vi "sub_main_state.vi"(8 "error in":errorcluster) -> (0 "error out":errorcluster)   [LabVIEW 2019]
uses:
  Ctrl/waypoint_buf.ctl
  Ctrl/state.ctl
  Ctrl/pid-in-params.ctl
  Ctrl/gps-databuf.ctl
panel:
  out "angle check":T1(graph)
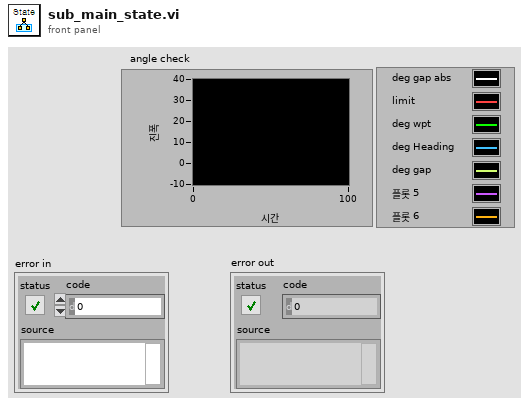
[diagram p1: front panel]
types:
  T1 = cluster{dbl, "adjust angle margin":dbl, "deg_waypoint":dbl, "Heading":dbl, dbl}
  T2 = typedef "waypoint_buf.ctl" = enum16{"clear", "write", "read"}
  T3 = typedef "state.ctl" = enum16{"init", "Test circular track", "start point", "start heading adjust", "wait before start", "stop point check", "stop point start", "end point", "entering ending point", "move", "move heading adjust"}
  T4 = typedef "pid-in-params.ctl" = enum16{"read", "write"}
  T5 = typedef "gps-databuf.ctl" = enum16{"read", "write"}
  T6 = cluster{"wpt group i":i32, "state total i":i32, "state main i":i32}
  T7 = cluster{"start point":cluster{"x":dbl, "y":dbl}, "stop point":cluster{"x":dbl, "y":dbl}}
  T8 = cluster{"lookahead pt n":dbl, "lookahead distance":dbl}
  T9 = cluster{"deg_agv-lookahead":dbl, "deg_waypoint":dbl, "deg_gap":dbl, "deg_target":dbl, "pid output":dbl, "dis-gap":dbl, "deg_agv-center":dbl}
  T10 = cluster{" turn angular speed":dbl, "move linear speed":dbl, "decrease factor linear speed":dbl, "adjust angle margin":dbl}
  T11 = cluster{"rawdata":string, "GPS Data":cluster{"Latitude":cluster{"Valid?":bool, "Latitude (Deg)":dbl}, "Longitude":cluster{"Valid?":bool, "Longitude (Deg)":dbl}, "Height":cluster{"Valid?":bool, "Height (m)":dbl}, "Undulation":cluster{"Valid?":bool, "Undulation(m)":dbl}, "North Vel":cluster{"Valid?":bool, "North Vel (m/s)":dbl}, "East Vel":cluster{"Valid?":bool, "East Vel (m/s)":dbl}, "Up Vel":cluster{"Valid?":bool, "Up Vel (m/s)":dbl}, "Roll":cluster{"Valid?":bool, "Roll (degrees)":dbl}, "Pitch":cluster{"Valid?":bool, "Pitch (degrees)":dbl}, "Azimuth":cluster{"Valid?":bool, "Azimuth (degrees)":dbl}, "Lat deviation":cluster{"Valid?":bool, "Lat deviation (m)":dbl}, "Long deviation":cluster{"Valid?":bool, "Long deviation (m)":dbl}, "Height deviation":cluster{"Valid?":bool, "Height deviation (m)":dbl}, "North vel deviation":cluster{"Valid?":bool, "North vel deviation (m/s)":dbl}, "East vel deviation":cluster{"Valid?":bool, "East vel deviation (m/s)":dbl}, "Up vel deviation":cluster{"Valid?":bool, "Up vel deviation (m/s)":dbl}, "Roll deviation":cluster{"Valid?":bool, "Roll deviation (degrees)":dbl}, "Pitch deviation":cluster{"Valid?":bool, "Pitch deviation (degrees)":dbl}, "Azimuth deviation":cluster{"Valid?":bool, "Azimuth deviation (degrees)":dbl}, "Ext sol status":cluster{"Valid?":bool, "Ext sol status":dbl}}, "Heading":dbl, "utm-1":cluster{"XN":dbl, "YE":dbl}}
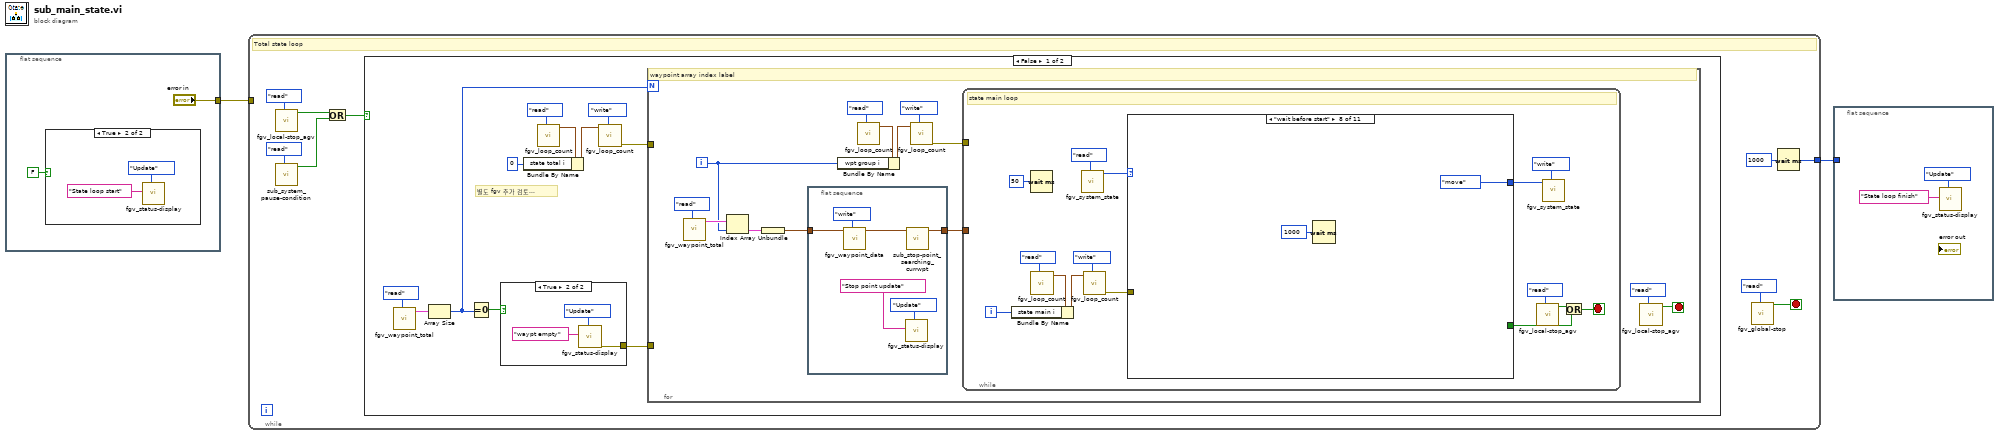
[diagram p0: block diagram]
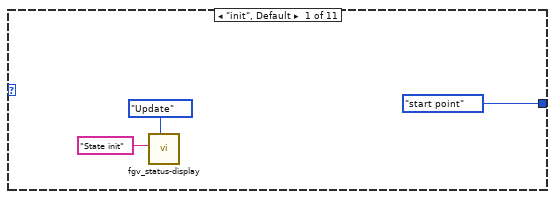
[diagram p4: hidden frame]
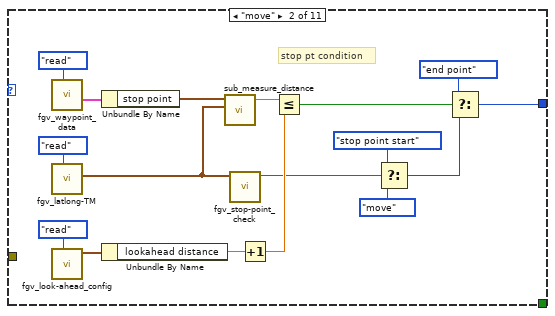
[diagram p5: hidden frame]
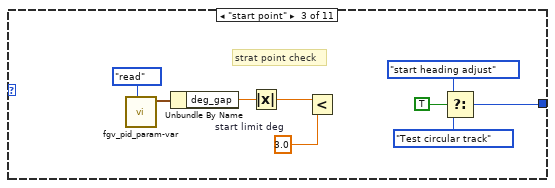
[diagram p6: hidden frame]
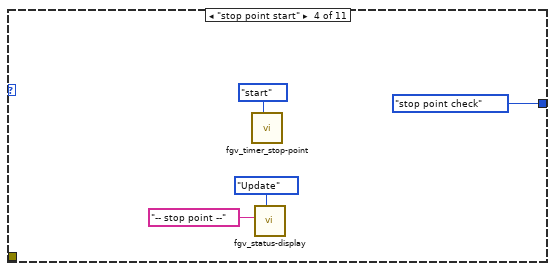
[diagram p7: hidden frame]
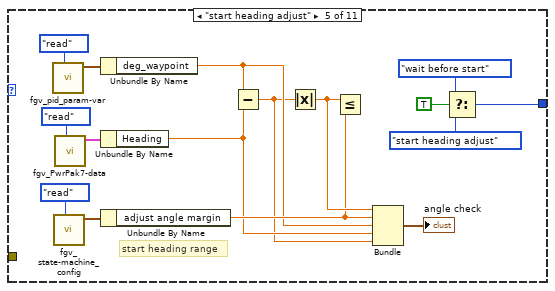
[diagram p8: hidden frame]
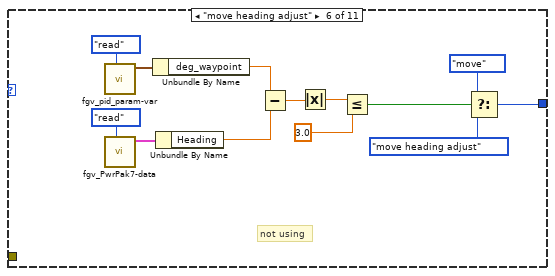
[diagram p9: hidden frame]
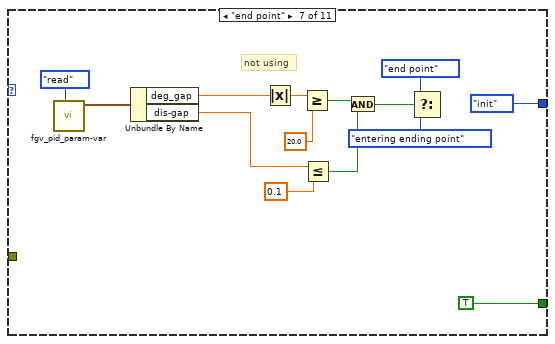
[diagram p10: hidden frame]
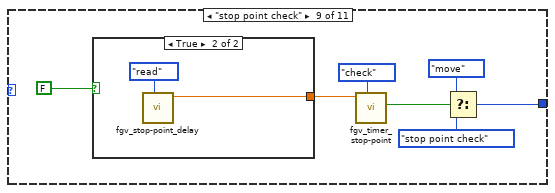
[diagram p11: hidden frame]
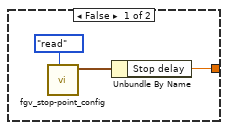
[diagram p12: hidden frame]
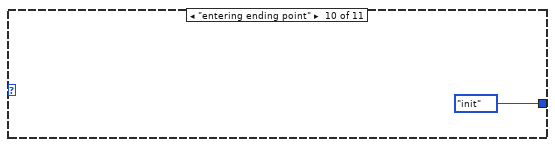
[diagram p13: hidden frame]
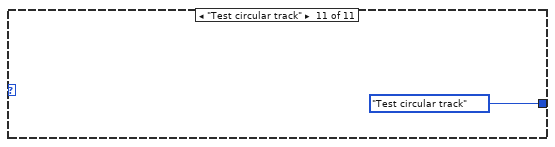
[diagram p14: hidden frame]
diagram:
  n1 = flat-sequence {
    tunnel: ["error in"] -> w2
    frame #0 {
      n2 = case shown="True" FALSE {
        frame False {
        }
        frame True {
          n3 = call "fgv_status-display.vi"("Mode"=enum16{"Initial", "Update", "Clear"}."Update", "title"="State loop start" ("String in 1")) -> ()  [unwired: 9 in, 1 out]
        }
      }
    }
  }
  n4 = while {
    tunnel: w2 -> [_]
    tunnel: [w14] -> w1
    stop <- w12 stop-if-true
    # "Total state loop"
    n5 = call "fgv_local-stop_agv.vi"("cmd"=enum16{"ini", "read", "stop"}."read") -> ("stop status"=w9:bool)  [unwired: 10 in]
    n6 = call "sub_system_pause-condition.vi"("cmd"=enum16{"pause", "go", "read"}."read") -> ("pause"=w7:bool)  [unwired: 10 in]
    n7 = Or(x=w9, y=w7) -> (x .or. y?=w8:bool)
    n8 = case shown="False" w8 {
      frame False {
        # "별도 fgv 추가 검토..."
        n9 = call "fgv_waypoint_total.vi"("cmd"=enum16{"write", "read"}."read") -> ("waypoint total out"=w24:cluster{"waypt":cluster{"X":dbl, "Y":dbl}[]}[])  [unwired: 10 in]
        n10 = Array Size(array=w24) -> (size(s)=w17:i32)
        n11 = Equal To 0?(x=w17) -> (x = 0?=w19:bool)
        n12 = case shown="True" w19 {
          tunnel: [_ w27] -> w26
          frame False {
          }
          frame True {
            n13 = call "fgv_status-display.vi"("Mode"=enum16{"Initial", "Update", "Clear"}."Update", "title"="waypt empty" ("String in 1")) -> ("error out"=w27:errorcluster)  [unwired: 9 in]
          }
        }
        n14 = call "fgv_loop_count.vi"("cmd"=enum16{"init", "read", "write"}."read") -> ("loop count out"=w21:T6)  [unwired: 9 in, 1 out]
        n15 = Bundle By Name(cluster=w21, "state total i"=0) -> (w20:T6)
        n16 = call "fgv_loop_count.vi"("cmd"=enum16{"init", "read", "write"}."write", "loop count in"=w20) -> ("error out"=w18:errorcluster)  [unwired: 8 in, 1 out]
        n17 = for {
          N: w17 -> [_]
          tunnel: w26 -> [_]
          tunnel: w18 -> [_]
          i -> [w32]
          stop <- w41 stop-if-true
          # "waypoint array index label"
          n18 = call "fgv_waypoint_total.vi"("cmd"=enum16{"write", "read"}."read") -> ("waypoint total out"=w33:cluster{"waypt":cluster{"X":dbl, "Y":dbl}[]}[])  [unwired: 10 in]
          n19 = Index Array(array=w33, index=w32) -> (element=w31:cluster{"waypt":cluster{"X":dbl, "Y":dbl}[]})
          n20 = Unbundle(w31) -> ("waypt"=w36:cluster{"X":dbl, "Y":dbl}[])
          n21 = flat-sequence {
            tunnel: w36 -> [w47]
            tunnel: [w43] -> w30
            frame #0 {
              n22 = call "fgv_waypoint_data.vi"("cmd"=waypoint_buf."write", "waypoint in"=w47) -> ("waypoint out"=w44:cluster{"x":dbl, "y":dbl}[])  [unwired: 7 in, 2 out]
              n23 = call "fgv_status-display.vi"("Mode"=enum16{"Initial", "Update", "Clear"}."Update", "title"="Stop point update" ("String in 1")) -> ()  [unwired: 9 in, 1 out]
              n24 = call "sub_stop-point_searching_currwpt.vi"("waypoint in"=w44) -> ("stop_point_buff"=w43:cluster{dbl, dbl}[])  [unwired: 10 in]
            }
          }
          n25 = call "fgv_loop_count.vi"("cmd"=enum16{"init", "read", "write"}."read") -> ("loop count out"=w38:T6)  [unwired: 9 in, 1 out]
          n26 = Bundle By Name(cluster=w38, "wpt group i"=w32) -> (w37:T6)
          n27 = call "fgv_loop_count.vi"("cmd"=enum16{"init", "read", "write"}."write", "loop count in"=w37) -> ("error out"=w35:errorcluster)  [unwired: 8 in, 1 out]
          n28 = while {
            tunnel: w35 -> [_]
            tunnel: w30 -> [_]
            i -> [w51]
            stop <- w60 stop-if-true
            # "state main loop"
            n29 = Wait (ms)(milliseconds to wait=u32 50 ("대기 시간 (ms)")) -> ()  [unwired: 1 out]
            n30 = call "fgv_loop_count.vi"("cmd"=enum16{"init", "read", "write"}."read") -> ("loop count out"=w53:T6)  [unwired: 9 in, 1 out]
            n31 = Bundle By Name(cluster=w53, "state main i"=w51) -> (w52:T6)
            n32 = call "fgv_system_state.vi"("cmd"=enum16{"init", "read", "write"}."read") -> ("State out"=w56:T3)  [unwired: 9 in, 1 out]
            n33 = call "fgv_loop_count.vi"("cmd"=enum16{"init", "read", "write"}."write", "loop count in"=w52) -> ("error out"=w50:errorcluster)  [unwired: 8 in, 1 out]
            n34 = case shown="\"wait before start\"" w56 {
              tunnel: [_ _ _ _ _ _ TRUE _ _ _ _] -> w58
              tunnel: [state."start point" ("f") w77 w90 state."stop point check" ("state") w111 w113 state."init" ("State out") state."move" ("state") w144 state."init" ("State out") state."Test circular track" ("State out")] -> w61
              tunnel: w50 -> [_ _ _ _ _ _ _ _ _ _ _]
              frame "init", Default {
                # "initial before start"
                n35 = call "fgv_status-display.vi"("Mode"=enum16{"Initial", "Update", "Clear"}."Update", "title"="State init" ("String in 1")) -> ()  [unwired: 9 in, 1 out]
              }
              frame "move" {
                # "stop pt condition"
                # "normal moving"
                n36 = call "fgv_waypoint_data.vi"("cmd"=waypoint_buf."read") -> ("start-stop point"=w80:T7)  [unwired: 8 in, 2 out]
                n37 = call "fgv_latlong-TM.vi"("cmd"=enum16{"write", "read"}."read") -> ("tm out"=w67:cluster{"YE":dbl, "XN":dbl})  [unwired: 9 in, 1 out]
                n38 = call "fgv_look-ahead_config.vi"("cmd"=enum16{"read", "write"}."read") -> ("lookahed cfg out"=w76:T8)  [unwired: 10 in]
                n39 = Unbundle By Name(w80) -> ("stop point"=w79:cluster{"x":dbl, "y":dbl})
                n40 = Unbundle By Name(w76) -> ("lookahead distance"=w75:dbl)
                n41 = call "sub_measure_distance.vi"("pt 2"=w67, "pt 1"=w79) -> ("distance"=w78:dbl)  [unwired: 9 in]
                n42 = call "fgv_stop-point_check.vi"("agv curr utm"=w67) -> ("stop point check"=w68:bool)  [unwired: 10 in]
                n43 = Increment(x=w75) -> (x+1=w74:dbl)
                n44 = Less Or Equal?(x=w78, y=w74) -> (x <= y?=w70:bool)
                n45 = Select(t=state."stop point start" ("state"), s=w68, f=state."move" ("state")) -> (s? t:f=w69:T3)
                n46 = Select(t=state."end point" ("state"), s=w70, f=w69) -> (s? t:f=w77:T3)
              }
              frame "start point" {
                w86 = 3.0  # start limit deg
                # "strat point check"
                n47 = call "fgv_pid_param-var.vi"("cmd"=pid-in-params."read") -> ("pid-var_output"=w88:T9)  [unwired: 10 in]
                n48 = Unbundle By Name(w88) -> ("deg_gap"=w87:dbl)
                n49 = Absolute Value(x=w87) -> (abs(x)=w85:dbl)
                n50 = Less?(x=w85, y=w86) -> ()  [unwired: 1 out]
                n51 = Select(t=state."start heading adjust" ("f"), s=TRUE, f=state."Test circular track") -> (s? t:f=w90:T3)
              }
              frame "stop point start" {
                n52 = call "fgv_timer_stop-point.vi"("cmd"=enum16{"check", "start", "pause"}."start") -> ()  [unwired: 8 in, 3 out]
                n53 = call "fgv_status-display.vi"("Mode"=enum16{"Initial", "Update", "Clear"}."Update", "title"="-- stop point --" ("String in 1")) -> ()  [unwired: 9 in, 1 out]
              }
              frame "start heading adjust" {
                # "start heading range"
                n54 = call "fgv_pid_param-var.vi"("cmd"=pid-in-params."read") -> ("pid-var_output"=w109:T9)  [unwired: 10 in]
                n55 = call "fgv_state-machine_config.vi"("cmd"=enum16{"write", "read"}."read") -> ("Angle cfg out"=w105:T10)  [unwired: 10 in]
                n56 = call "fgv_PwrPak7-data.vi"("cmd"=gps-databuf."read") -> ("data cluster out"=w108:T11)  [unwired: 9 in, 1 out]
                n57 = Unbundle By Name(w109) -> ("deg_waypoint"=w100:dbl)
                n58 = Unbundle By Name(w108) -> ("Heading"=w99:dbl)
                n59 = Unbundle By Name(w105) -> ("adjust angle margin"=w101:dbl)
                n60 = Subtract(x=w100, y=w99) -> (x-y=w98:dbl)
                n61 = Absolute Value(x=w98) -> (abs(x)=w102:dbl)
                n62 = Less Or Equal?(x=w102, y=w101) -> ()  [unwired: 1 out]
                n63 = Bundle(w102, "adjust angle margin"=w101, "deg_waypoint"=w100, "Heading"=w99, w98) -> (→"angle check":T1)  [unwired: 1 in]
                n64 = Select(t=state."wait before start" ("state"), s=TRUE, f=state."start heading adjust") -> (s? t:f=w111:T3)
              }
              frame "move heading adjust" {
                # "not using"
                n65 = call "fgv_pid_param-var.vi"("cmd"=pid-in-params."read") -> ("pid-var_output"=w123:T9)  [unwired: 10 in]
                n66 = call "fgv_PwrPak7-data.vi"("cmd"=gps-databuf."read") -> ("data cluster out"=w120:T11)  [unwired: 9 in, 1 out]
                n67 = Unbundle By Name(w123) -> ("deg_waypoint"=w118:dbl)
                n68 = Unbundle By Name(w120) -> ("Heading"=w117:dbl)
                n69 = Subtract(x=w118, y=w117) -> (x-y=w116:dbl)
                n70 = Absolute Value(x=w116) -> (abs(x)=w121:dbl)
                n71 = Less Or Equal?(x=w121, y=3.0) -> (x <= y?=w115:bool)
                n72 = Select(t=state."move" ("state"), s=w115, f=state."move heading adjust") -> (s? t:f=w113:T3)
              }
              frame "end point" {
                # "not using"
                n73 = call "fgv_pid_param-var.vi"("cmd"=pid-in-params."read") -> ("pid-var_output"=w132:T9)  [unwired: 10 in]
                n74 = Unbundle By Name(w132) -> ("deg_gap"=w133:dbl, "dis-gap"=w139:dbl)
                n75 = Absolute Value(x=w133) -> (abs(x)=w134:dbl)
                n76 = Greater Or Equal?(x=w134, y=20.0 ("angle adjust limit")) -> (x >= y?=w135:bool)
                n77 = Less Or Equal?(x=w139, y=0.1) -> (x <= y?=w136:bool)
                n78 = And(x=w135, y=w136) -> (x .and. y?=w137:bool)
                n79 = Select(t=state."end point" ("state"), s=w137, f=state."entering ending point") -> ()  [unwired: 1 out]
              }
              frame "wait before start" {
                n80 = Wait (ms)(milliseconds to wait=u32 1000) -> ()  [unwired: 1 out]
              }
              frame "stop point check" {
                n81 = case shown="True" FALSE {
                  tunnel: [w149 w152] -> w147
                  frame False {
                    n82 = call "fgv_stop-point_config.vi"("cmd"=enum16{"read", "write"}."read") -> ("config value out"=w150:cluster{"stop distance":dbl, "Stop delay":dbl})  [unwired: 10 in]
                    n83 = Unbundle By Name(w150) -> ("Stop delay"=w149:dbl)
                  }
                  frame True {
                    n84 = call "fgv_stop-point_delay.vi"("cmd"=enum16{"init", "read", "write"}."read") -> ("stop dt out"=w152:dbl)  [unwired: 9 in, 1 out]
                  }
                }
                n85 = call "fgv_timer_stop-point.vi"("cmd"=enum16{"check", "start", "pause"}."check", "target time"=w147) -> ("time-out"=w143:bool)  [unwired: 7 in, 2 out]
                n86 = Select(t=state."move" ("state"), s=w143, f=state."stop point check") -> (s? t:f=w144:T3)
              }
              frame "entering ending point" {
              }
              frame "Test circular track" {
              }
            }
            n87 = call "fgv_local-stop_agv.vi"("cmd"=enum16{"ini", "read", "stop"}."read") -> ("stop status"=w59:bool)  [unwired: 10 in]
            n88 = call "fgv_system_state.vi"("cmd"=enum16{"init", "read", "write"}."write", "State"=w61) -> ()  [unwired: 8 in, 2 out]
            n89 = Or(x=w59, y=w58) -> (x .or. y?=w60:bool)
          }
          n90 = call "fgv_local-stop_agv.vi"("cmd"=enum16{"ini", "read", "stop"}."read") -> ("stop status"=w41:bool)  [unwired: 10 in]
        }
      }
      frame True {
      }
    }
    n91 = call "fgv_global-stop.vi"("cmd"=enum16{"init", "stop", "read"}."read") -> ("val_out"=w12:bool)  [unwired: 10 in]
    n92 = Wait (ms)(milliseconds to wait=u32 1000) -> (millisecond timer value=w14:u32)
  }
  n93 = flat-sequence {
    tunnel: w1 -> [_]
    frame #0 {
      n94 = call "fgv_status-display.vi"("Mode"=enum16{"Initial", "Update", "Clear"}."Update", "title"="State loop finish" ("String in 1")) -> ()  [unwired: 9 in, 1 out]
    }
  }
